vi "Flow rate calc2.vi"(9 "T venturi":fxp<+/-,42,16> format="%.31g", 10 "P venturi":fxp<+/-,42,16> format="%.31g") -> (1 "Flow rate g/s":dbl, 2 "Flow rate l/min":dbl)   [LabVIEW 2014]
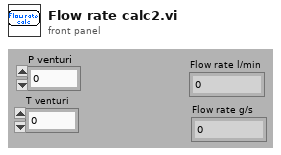
[diagram p1: front panel]
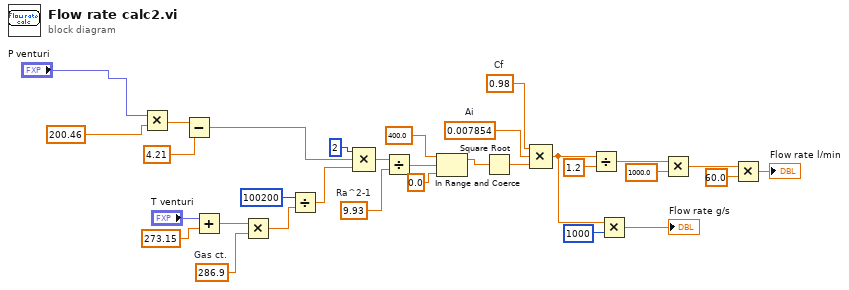
[diagram p0: block diagram]
diagram:
  w25 = 9.93  # Ra^2-1
  w22 = 0.98  # Cf
  w28 = 286.9  # Gas ct.
  w23 = 0.007854  # Ai
  n1 = Multiply(x="P venturi", y=200.46) -> (x*y=w4:dbl)
  n2 = Subtract(x=w4, y=4.21) -> (x-y=w2:dbl)
  n3 = Add(x="T venturi", y=273.15) -> (x+y=w29:dbl)
  n4 = Multiply(x=w29, y=w28) -> (x*y=w20:dbl)
  n5 = Divide(x=100200, y=w20) -> (x/y=w19:dbl)
  n6 = Compound Arithmetic op=MULTIPLY(2, w2, w19) -> (w26:dbl)
  n7 = Divide(x=w26, y=w25) -> (x/y=w9:dbl)
  n8 = In Range and Coerce(upper limit=400.0, x=w9, lower limit=0.0) -> (coerced(x)=w6:dbl)  [unwired: 1 out]
  n9 = Square Root(x=w6) -> (sqrt(x)=w24:dbl)
  n10 = Compound Arithmetic op=MULTIPLY(w22, w23, w24) -> (w16:dbl)
  n11 = Divide(x=w16, y=1.2) -> (x/y=w14:dbl)
  n12 = Multiply(x=w16, y=1000) -> (x*y=→"Flow rate g/s":dbl)
  n13 = Multiply(x=w14, y=1000.0) -> (x*y=w12:dbl)
  n14 = Multiply(x=w12, y=60.0) -> (x*y=→"Flow rate l/min":dbl)
